vi "_RT_CtrlLoop_Log writeFile.vi"(8 "error in":errorcluster, 10 "Describe":string) -> (0 "error out":errorcluster)   [LabVIEW 2018]
uses:
  <vilib>/Utility/file.llb/Write Delimited Spreadsheet (string).vi
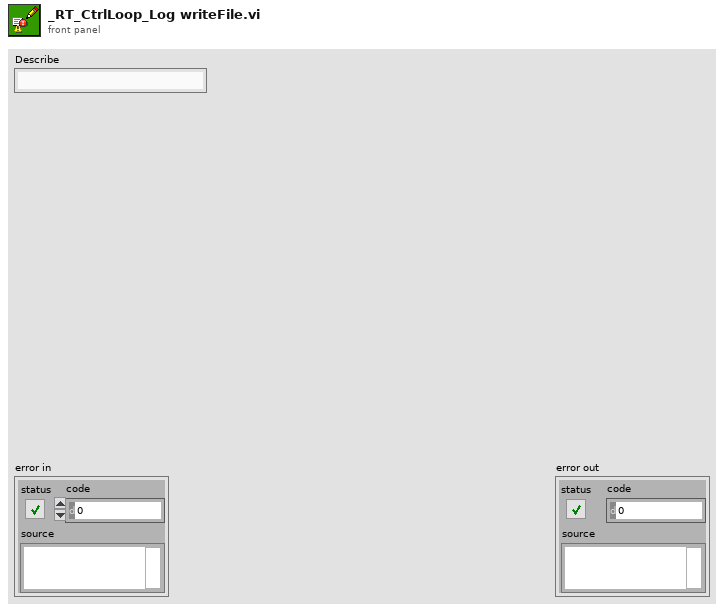
[diagram p1: front panel]
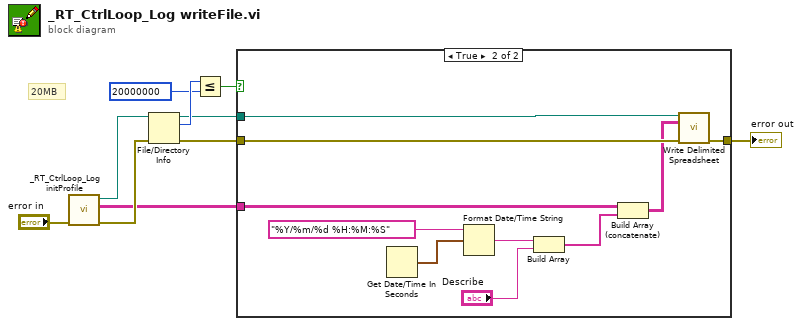
[diagram p0: block diagram]
diagram:
  # "20MB"
  n1 = call "_RT_CtrlLoop_Log initProfile.vi"("error in (no error)"="error in") -> ("error out"=w6:errorcluster, "all rows"=w1:string[][], "new file path"=w9:path)  [unwired: 8 in]
  n2 = File/Directory Info(path=w9, error in=w6) -> (path out=w4:path, size=w8:i64, error out=w3:errorcluster)  [unwired: 4 out]
  n3 = Less Or Equal?(x=w8, y=i64 20000000) -> (x <= y?=w5:bool)
  n4 = case shown="True" w5 {
    tunnel: w4 -> [_ w21]
    tunnel: w3 -> [w11 w20]
    tunnel: [w11 w19] -> w2
    tunnel: w1 -> [_ w17]
    frame False {
    }
    frame True {
      n5 = Get Date/Time In Seconds() -> (seconds since 1Jan1904=w18:timestamp)
      n6 = Format Date/Time String(time format string (%c)="%Y/%m/%d %H:%M:%S", seconds (now)=w18) -> (date/time string=w15:string)  [unwired: 1 in]
      n7 = Build Array(w15, "Describe") -> (w13:string[])
      n8 = Build Array (concatenate)(w17, w13) -> (w12:string[][])
      n9 = call-poly <vilib>:"Write Delimited Spreadsheet.vi"("file path (dialog if empty)"=w21, "2D data"=w12, "error in (no error)"=w20) -> ("error out"=w19:errorcluster)  [unwired: 11 in, 1 out]
    }
  }
  "error out" <- w2
